vi "Energia Create Build Cpp Command 2.vi"(10 "input filename":path=path "C:/Users/Simon Gurfunkel/Documents/LabVIEW_projects/LabVIEW-Universal-Transcriptor/Transcriptors/2/Examples - Arduino/Example_MSP430_Blink/blink.cpp", 11 "Code Composer directory":path=path "C:/ti/ccsv8") -> (1 "command load program into MCU":string, 2 "command to create .OUT":string, 3 "command to create .OBJ":string)   [LabVIEW 2018]
doc: "Create command to compile source code sketch for MSP340 Launchpad board.\n\nThis will create compile command to used compiler from Code Composer instead from Energia."
uses:
  <vilib>/regexp/Match Regular Expression.xnode
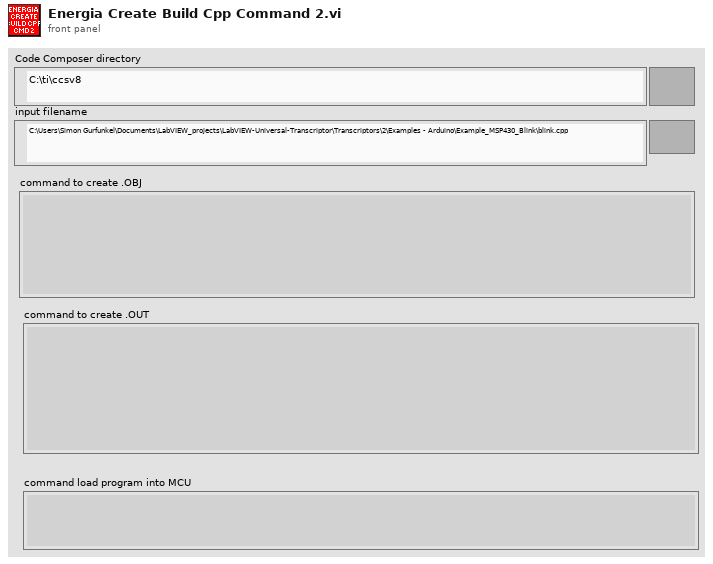
[diagram p1: front panel]
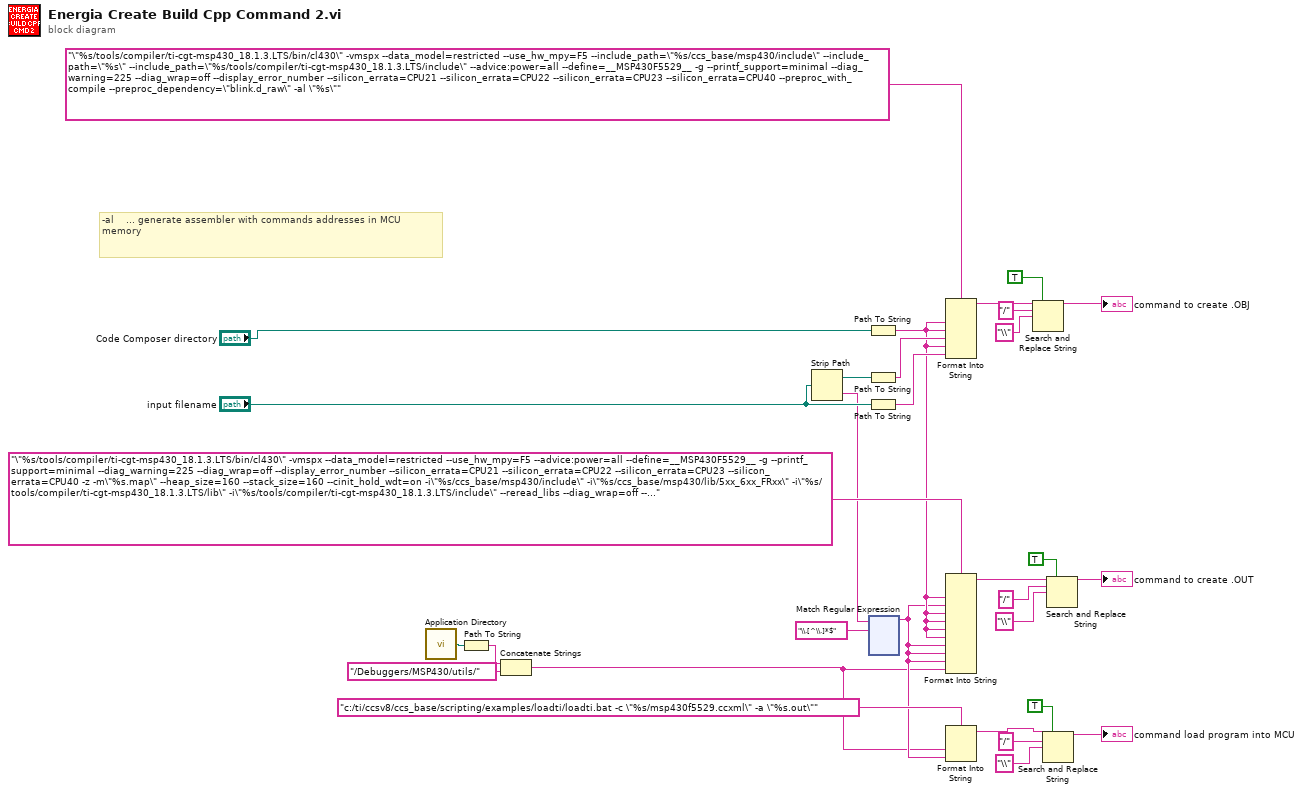
[diagram p0: block diagram]
diagram:
  # "-al    ... generate assembler with commands addresses in MCU memory"
  n1 = call <vilib>:"Application Directory.vi"() -> ("Application Directory"=w7:path)
  n2 = Path To String(path=w7) -> (string=w6:string)
  n3 = Concatenate Strings(w6, "/Debuggers/MSP430/utils/" ("string")) -> (w4:string)
  n4 = Strip Path(path="input filename") -> (stripped path=w31:path, name=w23:string)
  n5 = Path To String(path="Code Composer directory") -> (string=w22:string)
  n6 = Path To String(path=w31) -> (string=w29:string)
  n7 = Path To String(path="input filename") -> (string=w27:string)
  n8 = xnode ("Match Regular Expression")("input string"=w23, "regular expression"="\\.[^\\.]*$" ("input string")) -> ("before match"=w20:string)  [unwired: 4 in, 4 out]
  n9 = Format Into String(format string="\"%s/tools/compiler/ti-cgt-msp430_18.1.3.LTS/bin/cl430\" -vmspx --data_model=restricted --use_hw_mpy=F5 --include_path=\"%s/ccs_base/msp430/include\" --include_path=\"%s\" --include_path=\"%s/tools/compiler/ti-cgt-msp430_18.1.3.LTS/include\" --advice:power=all --define=__MSP430F5529__ -g --printf_support=minimal --diag_warning=225 --diag_wrap=off --display_error_number --silicon_errata=CPU21 --silicon_errata=CPU22 --silicon_errata=CPU23 --silicon_errata=CPU40 --preproc_with_compile --preproc_dependency=\"blink.d_raw\" -al \"%s\"", w22, w22, w29, w22, w27) -> (resulting string=w19:string)  [unwired: 2 in, 1 out]
  n10 = Format Into String(format string="\"%s/tools/compiler/ti-cgt-msp430_18.1.3.LTS/bin/cl430\" -vmspx --data_model=restricted --use_hw_mpy=F5 --advice:power=all --define=__MSP430F5529__ -g --printf_support=minimal --diag_warning=225 --diag_wrap=off --display_error_number --silicon_errata=CPU21 --silicon_errata=CPU22 --silicon_errata=CPU23 --silicon_errata=CPU40 -z -m\"%s.map\" --heap_size=160 --stack_size=160 --cinit_hold_wdt=on -i\"%s/ccs_base/msp430/include\" -i\"%s/ccs_base/msp430/lib/5xx_6xx_FRxx\" -i\"%s/tools/compiler/ti-cgt-msp430_18.1.3.LTS/lib\" -i\"%s/tools/compiler/ti-cgt-msp430_18.1.3.LTS/include\" --reread_libs --diag_wrap=off --display_error_number --warn_sections --xml_link_info=\"%s_linkInfo.xml\" --use_hw_mpy=F5 --rom_model -o \"%s.out\" \"./%s.obj\" \"%s/lnk_msp430f5529.cmd\"  -llibmath.a -llibc.a", w22, w20, w22, w22, w22, w22, w20, w20, w20, w4) -> (resulting string=w10:string)  [unwired: 2 in, 1 out]
  n11 = Format Into String(format string="c:/ti/ccsv8/ccs_base/scripting/examples/loadti/loadti.bat -c \"%s/msp430f5529.ccxml\" -a \"%s.out\"" ("input string"), w4, w20) -> (resulting string=w11:string)  [unwired: 2 in, 1 out]
  n12 = Search and Replace String(replace all?=TRUE ("replace all? (F)"), input string=w19, search string="/", replace string="\\" ("search string")) -> (result string=→"command to create .OBJ":string)  [unwired: 4 in, 3 out]
  n13 = Search and Replace String(replace all?=TRUE ("replace all? (F)"), input string=w11, search string="/", replace string="\\" ("search string")) -> (result string=→"command load program into MCU":string)  [unwired: 4 in, 3 out]
  n14 = Search and Replace String(replace all?=TRUE ("replace all? (F)"), input string=w10, search string="/", replace string="\\" ("search string")) -> (result string=→"command to create .OUT":string)  [unwired: 4 in, 3 out]
